vi "PHD2000 manual control.vi"(8 "error in (no error)":errorcluster, 9 "Pump #":string="0", 10 "control":T1 {"Target volume (ml)" min=0.0 max=50.0 format="%#.3g"; "Flowrate (ml/min)" min=0.0 max=500.0 format="%#.3g"}, 11 "VISA resource name 2":refnum<visa-resource-name>) -> (0 "error out":errorcluster, 3 "VISA resource name out":refnum<visa-resource-name>)   [LabVIEW 2017]
uses:
  <instrlib>/Harvard Syringe Pump PHD2000/Harvard Syringe Pump PHD2000.lvlib
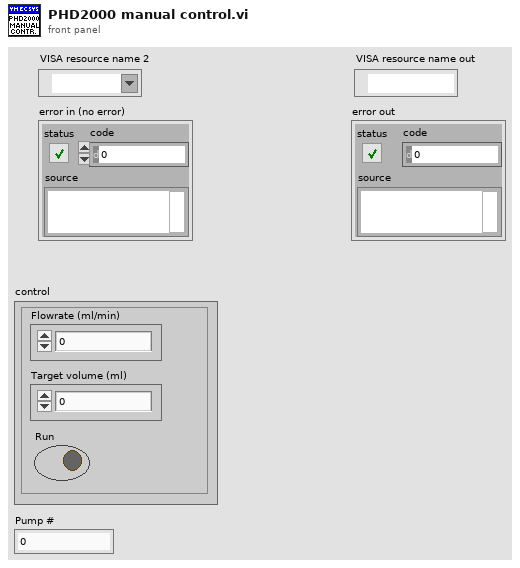
[diagram p1: front panel]
types:
  T1 = cluster{"Flowrate (ml/min)":dbl, "Target volume (ml)":dbl, "Run":bool}
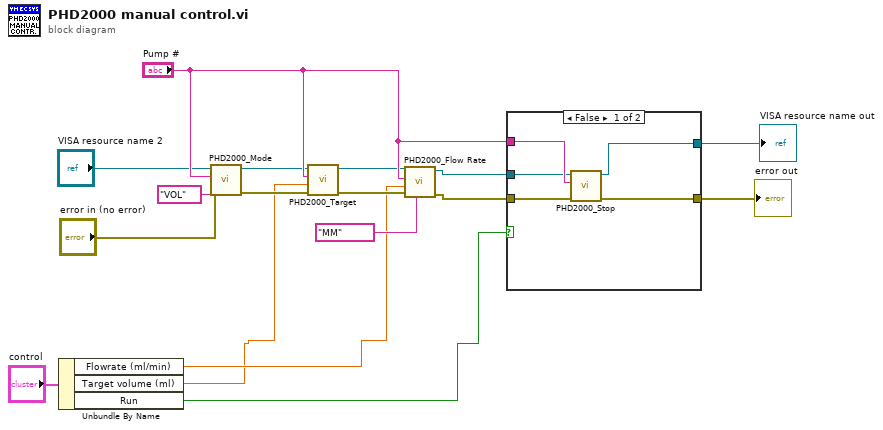
[diagram p0: block diagram]
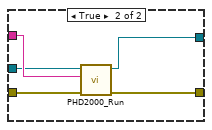
[diagram p2: hidden frame]
diagram:
  n1 = Unbundle By Name("control") -> ("Flowrate (ml/min)"=w3:dbl, "Target volume (ml)"=w2:dbl, "Run"=w1:bool)
  n2 = call <instrlib>:"PHD2000_Mode.vi"("error in (no error)"="error in (no error)", "Mode"="VOL", "Pump #"="Pump #", "VISA resource name 2"="VISA resource name 2") -> ("error out"=w9:errorcluster, "VISA resource name out"=w16:refnum<visa-resource-name>)  [unwired: 5 in, 1 out]
  n3 = call <instrlib>:"PHD2000_Target.vi"("error in (no error)"=w9, "Target (ml)"=w2, "Pump #"="Pump #", "VISA resource name 2"=w16) -> ("error out"=w8:errorcluster, "VISA resource name out"=w15:refnum<visa-resource-name>)  [unwired: 5 in, 1 out]
  n4 = call <instrlib>:"PHD2000_Flow Rate.vi"("VISA resource name 2"=w15, "Pump #"="Pump #", "flowrate"=w3, "error in (no error)"=w8, "Unit"="MM") -> ("VISA resource name out"=w14:refnum<visa-resource-name>, "error out"=w12:errorcluster)  [unwired: 4 in]
  n5 = case shown="False" w1 {
    tunnel: "Pump #" -> [w22 w27]
    tunnel: w14 -> [w18 w26]
    tunnel: w12 -> [w19 w25]
    tunnel: [w20 w24] -> w11
    tunnel: [w21 w23] -> w10
    frame False {
      n6 = call <instrlib>:"PHD2000_Stop.vi"("VISA resource name 2"=w18, "Pump #"=w22, "error in (no error)"=w19) -> ("VISA resource name out"=w21:refnum<visa-resource-name>, "error out"=w20:errorcluster)  [unwired: 6 in]
    }
    frame True {
      n7 = call <instrlib>:"PHD2000_Run.vi"("VISA resource name 2"=w26, "Pump #"=w27, "error in (no error)"=w25) -> ("VISA resource name out"=w23:refnum<visa-resource-name>, "error out"=w24:errorcluster)  [unwired: 6 in]
    }
  }
  "error out" <- w11
  "VISA resource name out" <- w10
